vi "Calculate Image Quality.vi"(8 "error in (no error)":errorcluster, 9 "Image Pixels to Compare (U32)":u32[][](array[numeric]), 10 "Image to Compare":T1, 11 "Expected Image":T1) -> (0 "error out":errorcluster, 3 "Quality":dbl format="%0.2f")   [LabVIEW 2023]
uses:
  <vilib>/vision/Image Controls.llb/IMAQ Image.ctl
panel:
  # "Overview:  Use this helper VI to compare images. It doesn't use any Vision Development Module functions to compare the image so no additional toolkits are required with this VI.\n\nExpected Image: The image that is expected. This comes from the acquisition and will be compared against images read from file to see if it's an exact match.\nImage to Compare: A reference to the image read from file to compare against the Expected Image. This input is only used when an image is wired into this input.\nImage Pixels to Compare (U32): The 2D array of pixel data read from a file to compare against the Expected Image. This input is only used when no image is wired into the Image to Compare input.\nQuality: An indication of the image quality. This currently does a simple equality test and returns 1 if the images are equal and 0 if they are not. You could add the Vision Development Module's SSIM algorithm comparison to get a more accurate measure of the quality and this also returns 1 for a perfect match and 0 for a poor match, but it will have values in between to indicate how closely they match if it's not a perfect match."
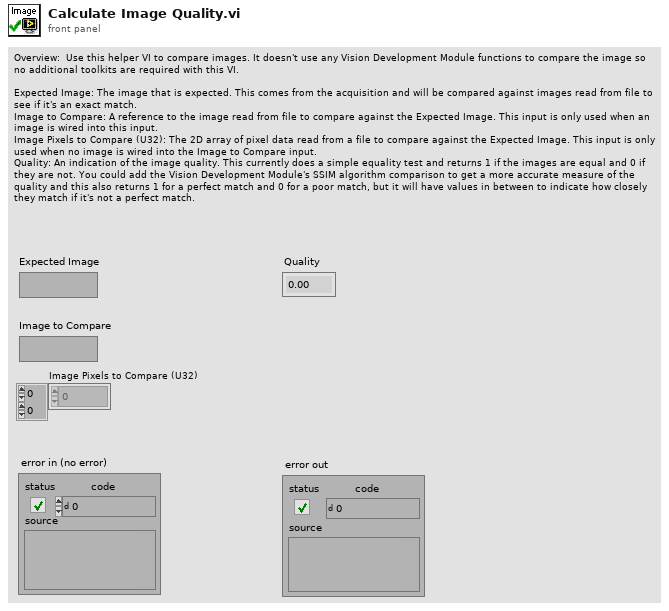
[diagram p1: front panel]
types:
  T1 = typedef "IMAQ Image.ctl" = refnum<image>
  T2 = typedef "Image Type" = u32
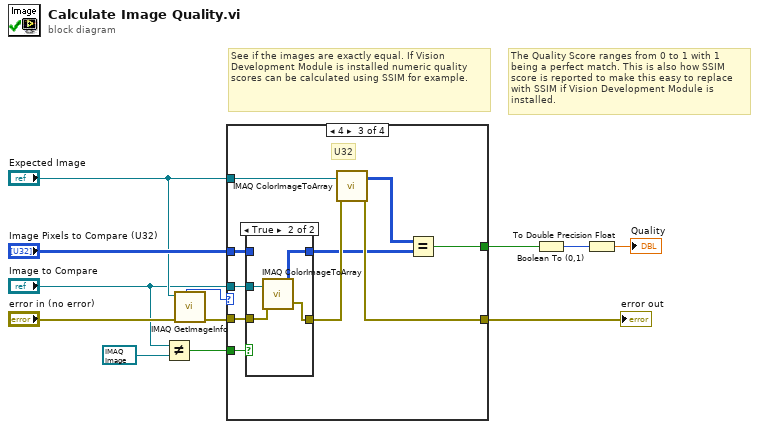
[diagram p0: block diagram]
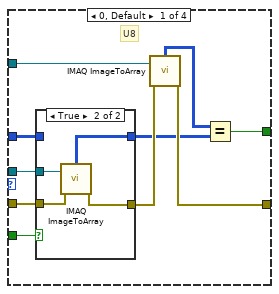
[diagram p2: hidden frame]
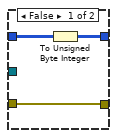
[diagram p3: hidden frame]
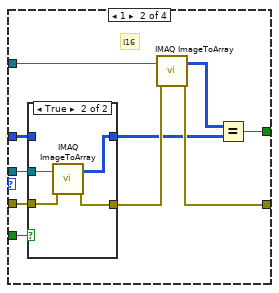
[diagram p4: hidden frame]
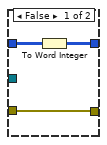
[diagram p5: hidden frame]
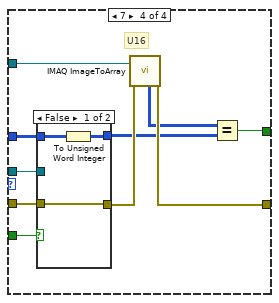
[diagram p7: hidden frame]
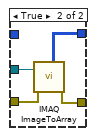
[diagram p8: hidden frame]
diagram:
  # "See if the images are exactly equal. If Vision Development Module is installed numeric quality scores can be calculated using SSIM for example."
  # "The Quality Score ranges from 0 to 1 with 1 being a perfect match. This is also how SSIM score is reported to make this easy to replace with SSIM if Vision Development Module is installed."
  n1 = Not Equal?(x="Image to Compare", y=T1 refnum) -> (x != y?=w1:bool)
  n2 = call "IMAQ GetImageInfo"("error in (no error)"="error in (no error)", "Image"="Expected Image") -> ("error out"=w5:errorcluster, "Image Type"=w4:T2)  [unwired: 2 in, 6 out]
  n3 = case shown="4" w4 {
    tunnel: "Expected Image" -> [w18 w35 w52 w68]
    tunnel: "Image Pixels to Compare (U32)" -> [w20 w39 w55 w69]
    tunnel: "Image to Compare" -> [w22 w37 w54 w71]
    tunnel: w1 -> [w21 w38 w56 w72]
    tunnel: w5 -> [w19 w36 w53 w70]
    tunnel: [w16 w33 w50 w66] -> w11
    tunnel: [w13 w30 w47 w63] -> w10
    frame 0, Default {
      # "U8"
      n4 = case shown="True" w21 {
        tunnel: w22 -> [_ w29]
        tunnel: [w24 w28] -> w15
        tunnel: w20 -> [w25 _]
        tunnel: w19 -> [w23 w27]
        tunnel: [w23 w26] -> w17
        frame False {
          n5 = To Unsigned Byte Integer(number=w25) -> (unsigned 8bit integer=w24:u8[][])
        }
        frame True {
          n6 = call "IMAQ ImageToArray"("error in (no error)"=w27, "Image"=w29) -> ("error out"=w26:errorcluster, "Image Pixels (U8)"=w28:u8[][])  [unwired: 2 in, 3 out]
        }
      }
      n7 = call "IMAQ ImageToArray"("error in (no error)"=w17, "Image"=w18) -> ("error out"=w16:errorcluster, "Image Pixels (U8)"=w14:u8[][])  [unwired: 2 in, 3 out]
      n8 = Equal?(x=w14, y=w15) -> (x = y?=w13:bool)
    }
    frame 1 {
      # "I16"
      n9 = case shown="True" w38 {
        tunnel: w39 -> [w42 _]
        tunnel: [w41 w43] -> w31
        tunnel: w37 -> [_ w46]
        tunnel: w36 -> [w40 w45]
        tunnel: [w40 w44] -> w34
        frame False {
          n10 = To Word Integer(number=w42) -> (16bit integer=w41:i16[][])
        }
        frame True {
          n11 = call "IMAQ ImageToArray"("error in (no error)"=w45, "Image"=w46) -> ("error out"=w44:errorcluster, "Image Pixels (I16)"=w43:i16[][])  [unwired: 2 in, 3 out]
        }
      }
      n12 = call "IMAQ ImageToArray"("error in (no error)"=w34, "Image"=w35) -> ("error out"=w33:errorcluster, "Image Pixels (I16)"=w32:i16[][])  [unwired: 2 in, 3 out]
      n13 = Equal?(x=w32, y=w31) -> (x = y?=w30:bool)
    }
    frame 4 {
      # "U32"
      n14 = case shown="True" w56 {
        tunnel: w55 -> [w58 _]
        tunnel: [w58 w60] -> w49
        tunnel: w54 -> [_ w62]
        tunnel: w53 -> [w57 w61]
        tunnel: [w57 w59] -> w51
        frame False {
        }
        frame True {
          n15 = call "IMAQ ColorImageToArray"("Image"=w62, "error in (no error)"=w61) -> ("Image Pixels (U32)"=w60:u32[][], "error out"=w59:errorcluster)  [unwired: 2 in, 1 out]
        }
      }
      n16 = call "IMAQ ColorImageToArray"("Image"=w52, "error in (no error)"=w51) -> ("Image Pixels (U32)"=w48:u32[][], "error out"=w50:errorcluster)  [unwired: 2 in, 1 out]
      n17 = Equal?(x=w48, y=w49) -> (x = y?=w47:bool)
    }
    frame 7 {
      # "U16"
      n18 = case shown="False" w72 {
        tunnel: w71 -> [_ w79]
        tunnel: w70 -> [w73 w78]
        tunnel: [w73 w77] -> w67
        tunnel: [w74 w76] -> w65
        tunnel: w69 -> [w75 _]
        frame False {
          n19 = To Unsigned Word Integer(number=w75) -> (unsigned 16bit integer=w74:u16[][])
        }
        frame True {
          n20 = call "IMAQ ImageToArray"("error in (no error)"=w78, "Image"=w79) -> ("Image Pixels (U16)"=w76:u16[][], "error out"=w77:errorcluster)  [unwired: 2 in, 3 out]
        }
      }
      n21 = call "IMAQ ImageToArray"("error in (no error)"=w67, "Image"=w68) -> ("Image Pixels (U16)"=w64:u16[][], "error out"=w66:errorcluster)  [unwired: 2 in, 3 out]
      n22 = Equal?(x=w64, y=w65) -> (x = y?=w63:bool)
    }
  }
  "error out" <- w11
  n23 = Boolean To (0,1)(Boolean=w10) -> (0, 1=w9:i16)
  n24 = To Double Precision Float(number=w9) -> (double precision float=→"Quality":dbl)
